vi "Create.vi"(8 "error in (no error)":errorcluster, 10 "Port":dbl=27015.0, 11 "Address":string="localhost") -> (0 "error out":errorcluster, 3 "TecellaClient out":refnum<class "TecellaClient.lvclass">)   [LabVIEW 2009, in "TecellaClient.lvclass"]
uses:
  TecellaClient.lvclass
  TecellaClient.lvclass/TecellaClient.ctl
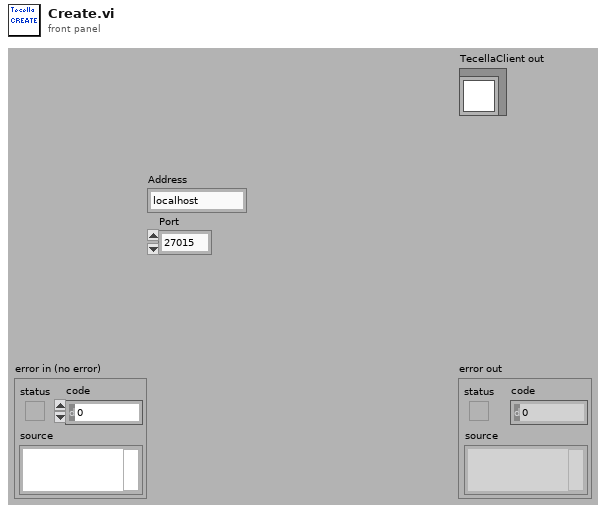
[diagram p1: front panel]
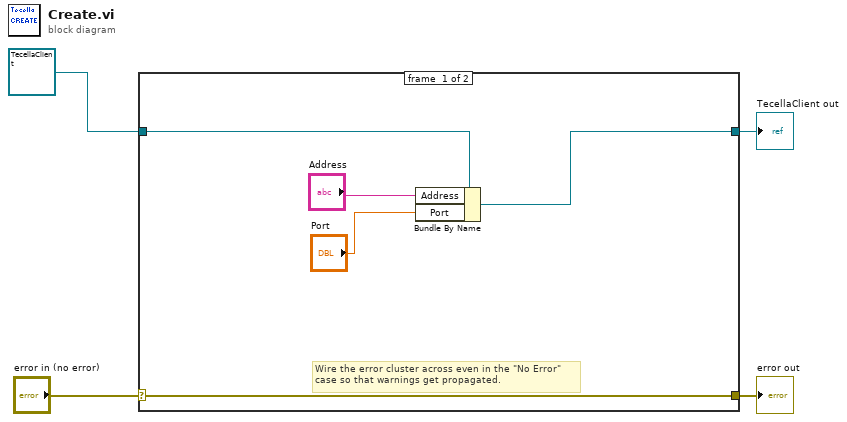
[diagram p0: block diagram]
diagram:
  n1 = case shown="No Error" "error in (no error)" {
    selector: "error in (no error)" -> [w9 w11]
    tunnel: [w9 w11] -> w3
    tunnel: [w5 w10] -> w1
    tunnel: refnum<class "TecellaClient.lvclass"> refnum ("TecellaClient in") -> [w6 w10]
    frame #0 {
      # "Wire the error cluster across even in the \"No Error\"\ncase so that warnings get propagated."
      n2 = Bundle By Name(cluster=w6, "Address"="Address", "Port"="Port") -> (w5:refnum<class "TecellaClient.lvclass">)
    }
    frame #1 {
    }
  }
  "error out" <- w3
  "TecellaClient out" <- w1
